vi "Write type.vi"(8 "error in (no error)":errorcluster, 10 "type":string, 11 "Start Calibration MSG in":refnum<class "Start Calibration MSG.lvclass">) -> (0 "error out":errorcluster, 3 "Start Calibration MSG out":refnum<class "Start Calibration MSG.lvclass">)   [LabVIEW 2014, in "Controller.lvlib" / "Start Calibration MSG.lvclass"]
uses:
  Start Calibration MSG.lvclass
  Start Calibration MSG.lvclass/Start Calibration MSG.ctl
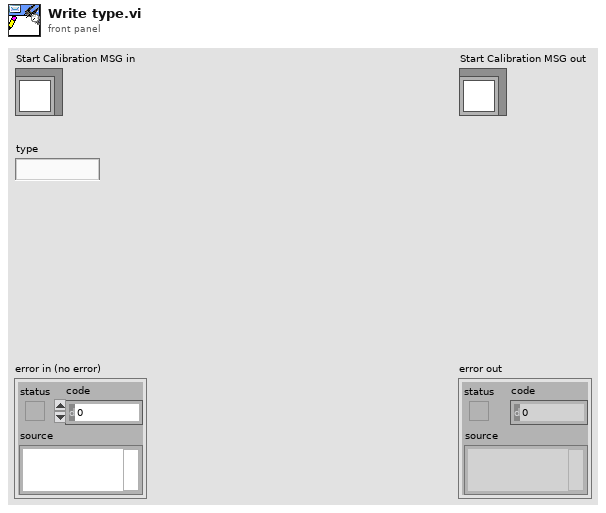
[diagram p1: front panel]
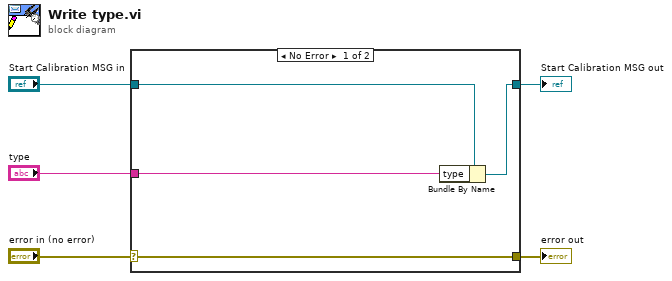
[diagram p0: block diagram]
diagram:
  n1 = case shown="No Error" "error in (no error)" {
    selector: "error in (no error)" -> [w9 w10]
    tunnel: [w9 w10] -> w4
    tunnel: [w7 w11] -> w2
    tunnel: "Start Calibration MSG in" -> [w8 w11]
    tunnel: "type" -> [w6 _]
    frame No Error {
      n2 = Bundle By Name(cluster=w8, "type"=w6) -> (w7:refnum<class "Start Calibration MSG.lvclass">)
    }
    frame Error {
    }
  }
  "error out" <- w4
  "Start Calibration MSG out" <- w2
